vi "motorStop.vi"(3 "error in (no error)":errorcluster, 5 "UART PORT in":refnum<visa-resource-name>) -> (0 "error out":errorcluster, 1 "P1":dbl[](array[numeric]), 2 "UART PORT out":refnum<visa-resource-name>)   [LabVIEW 2016]
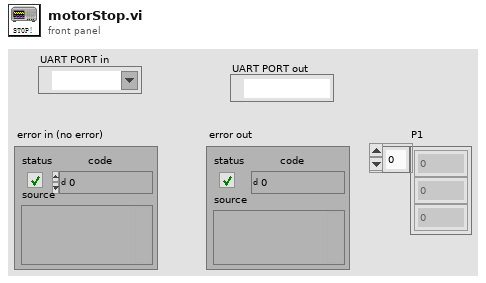
[diagram p1: front panel]
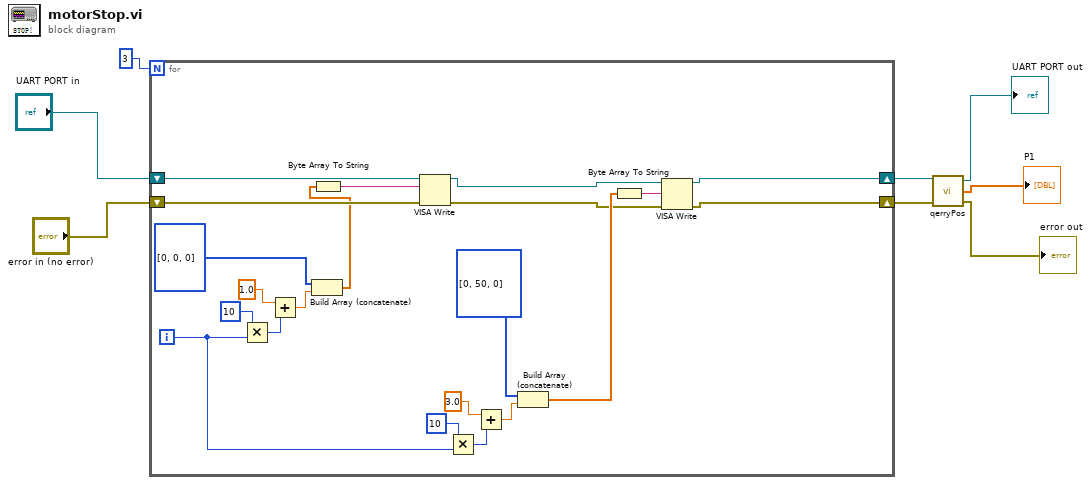
[diagram p0: block diagram]
diagram:
  n1 = for {
    N: 3 -> [_]
    shift-right: [w20] -> w8
    shift-left: "error in (no error)" -> [w28]
    shift-right: [w19] -> w7
    shift-left: "UART PORT in" -> [w27]
    i -> [w14]
    n2 = Multiply(x=10, y=w14) -> (x*y=w25:i32)
    n3 = Add(x=1.0, y=w25) -> (x+y=w21:dbl)
    n4 = Build Array (concatenate)(i32[] [0, 0, 0], w21) -> (w22:dbl[])
    n5 = Byte Array To String(unsigned byte array=w22) -> (string=w29:string)
    n6 = VISA Write(VISA resource name=w27, write buffer=w29, error in (no error)=w28) -> (VISA resource name out=w10:refnum<visa-resource-name>, error out=w9:errorcluster)  [unwired: 1 out]
    n7 = Multiply(x=10, y=w14) -> (x*y=w17:i32)
    n8 = Add(x=3.0, y=w17) -> (x+y=w15:dbl)
    n9 = Build Array (concatenate)(i32[] [0, 50, 0], w15) -> (w11:dbl[])
    n10 = Byte Array To String(unsigned byte array=w11) -> (string=w12:string)
    n11 = VISA Write(VISA resource name=w10, write buffer=w12, error in (no error)=w9) -> (VISA resource name out=w19:refnum<visa-resource-name>, error out=w20:errorcluster)  [unwired: 1 out]
  }
  n12 = call "qerryPos.vi"("error in (no error)"=w8, "UART in"=w7) -> ("error out"=→"error out":errorcluster, "Array"=→"P1":dbl[], "UART out"=→"UART PORT out":refnum<visa-resource-name>)  [unwired: 2 in]
